vi "FXP NILIA_DetectFrequency.vi"(9 "set":bool, 11 "x":fxp<+/-,24,1>) -> (1 "f_2":fxp<+/-,32,0> format="%.32g", 3 "f":fxp<+/-,32,0> format="%.32g")   [LabVIEW 2012]
uses:
  <vilib>/rvi/FXPMathLib/FxpDiv/subVIs/nifxpmath_Div_SimConfig.ctl
  <vilib>/rvi/FXPMathLib/FxpDiv/simVIs/DllFxpDivTemp_sub.vi
  <vilib>/rvi/FXPMathLib/FxpReciprocal/XNode/nifxpmath_Reciprocal.xnode
  <vilib>/rvi/FXPMathLib/FxpDiv/XNode/nifxpmath_Div.xnode
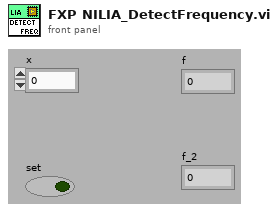
[diagram p1: front panel]
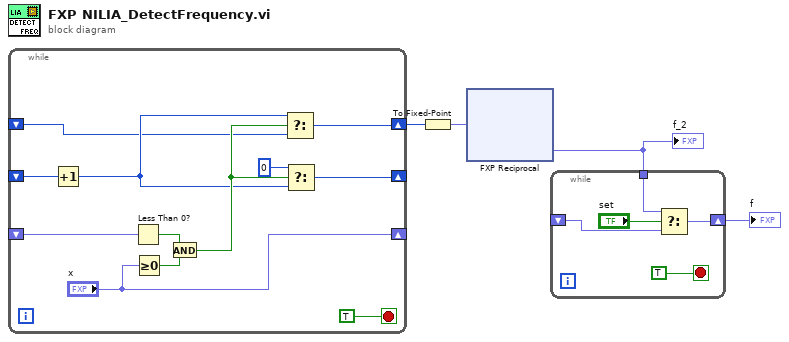
[diagram p0: block diagram]
diagram:
  n1 = while {
    shift-right: ["x"] -> _
    shift-left: _ -> [w16]
    shift-right: [w11] -> _
    shift-left: _ -> [w10]
    shift-right: [w7] -> w4
    shift-left: _ -> [w6]
    stop <- TRUE stop-if-true
    n2 = Increment(x=w10) -> (x+1=w8:i32)
    n3 = Less Than 0?(x=w16) -> (x < 0?=w14:bool)
    n4 = Greater Or Equal To 0?(x="x") -> (x >= 0?=w13:bool)
    n5 = And(x=w14, y=w13) -> (x .and. y?=w9:bool)
    n6 = Select(t=w8, s=w9, f=w6) -> (s? t:f=w7:i32)
    n7 = Select(t=0, s=w9, f=w8) -> (s? t:f=w11:i32)
  }
  n8 = To Fixed-Point(number=w4) -> (fixed-point=w3:fxp<+/-,32,32>)  [unwired: 1 in]
  n9 = xnode "FXP Reciprocal"("x"=w3) -> ("1/x"=w2:fxp<+/-,32,0>)
  "f_2" <- w2
  n10 = while {
    shift-right: [w18] -> w1
    shift-left: _ -> [w17]
    tunnel: w2 -> [w19]
    stop <- TRUE stop-if-true
    n11 = Select(t=w19, s="set", f=w17) -> (s? t:f=w18:fxp<+/-,32,0>)
  }
  "f" <- w1
